vi "PSFormula_Formula Node Generation.vi"(6 "Complex Variable(T)":bool=TRUE, 10 "Var List":T1={"Names"=["d", "r"], "Types"=["Array Of Dbl", "Dbl"], "Values"=[variant(dbl[] [0.0, 1.0]), variant(dbl 5.0)]}, 11 "Fomula":string="d+((d+r)*(4+5)+7)*8") -> (0 "Error Code":i32, 3 "Formula Node":T2)   [LabVIEW 2016]
uses:
  Ctrls/PSFormula_FOR_Formula Node.ctl
  Ctrls/PSFormula_FOR_Formula Step.ctl
  Ctrls/PSFormula_FOR_Formula Para.ctl
  Ctrls/PSFormula_FOR_Formula MidVar Data.ctl
panel:
  out "Numeric":i32
  out "Fomulas In Bracket":string[](array[string])
  # "d+((d+r)*(4+5)+7)*8"
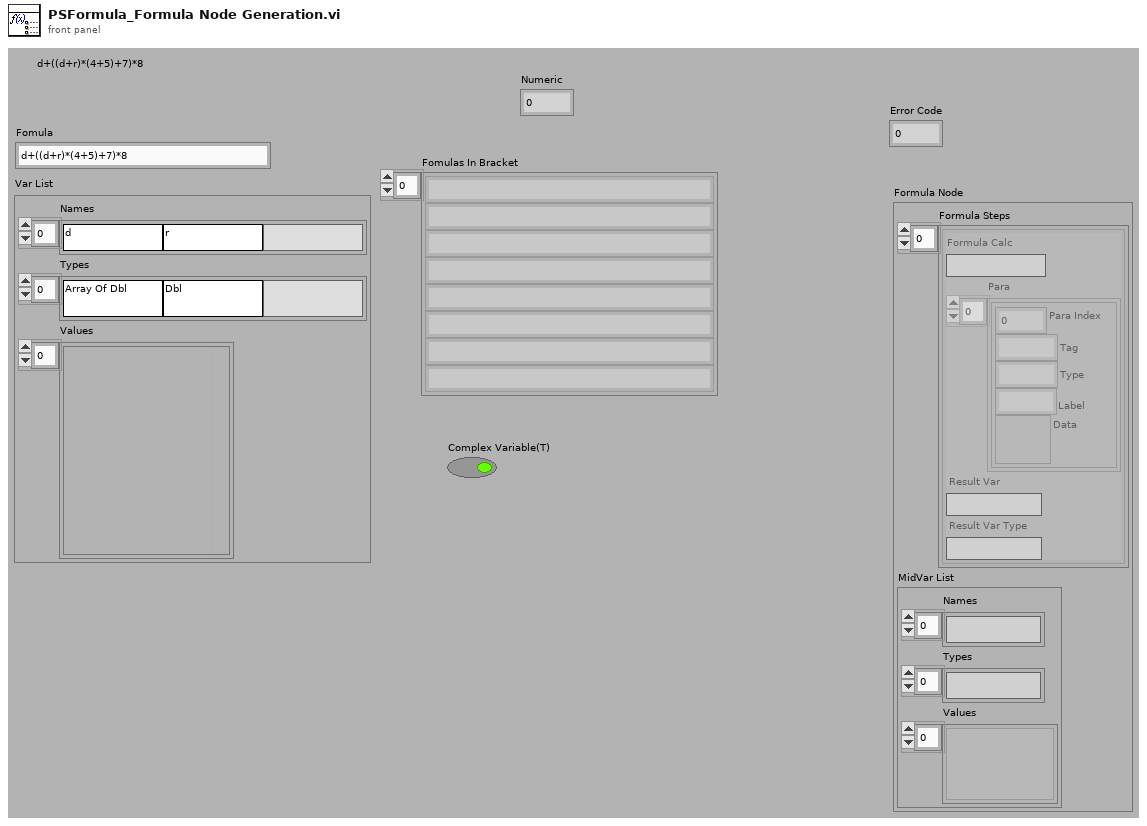
[diagram p1: front panel]
types:
  T1 = typedef "PSFormula_FOR_Formula MidVar Data.ctl" = cluster{"Names":string[], "Types":string[], "Values":variant[]}
  T2 = typedef "PSFormula_FOR_Formula Node.ctl" = cluster{"Formula Steps":T3[], "MidVar List":T1}
  T3 = typedef "PSFormula_FOR_Formula Step.ctl" = cluster{"Formula Calc":string, "Para":T4[], "Result Var":string, "Result Var Type":string}
  T4 = typedef "PSFormula_FOR_Formula Para.ctl" = cluster{"Para Index":i32, "Tag":string, "Type":string, "Label":string, "Data":variant}
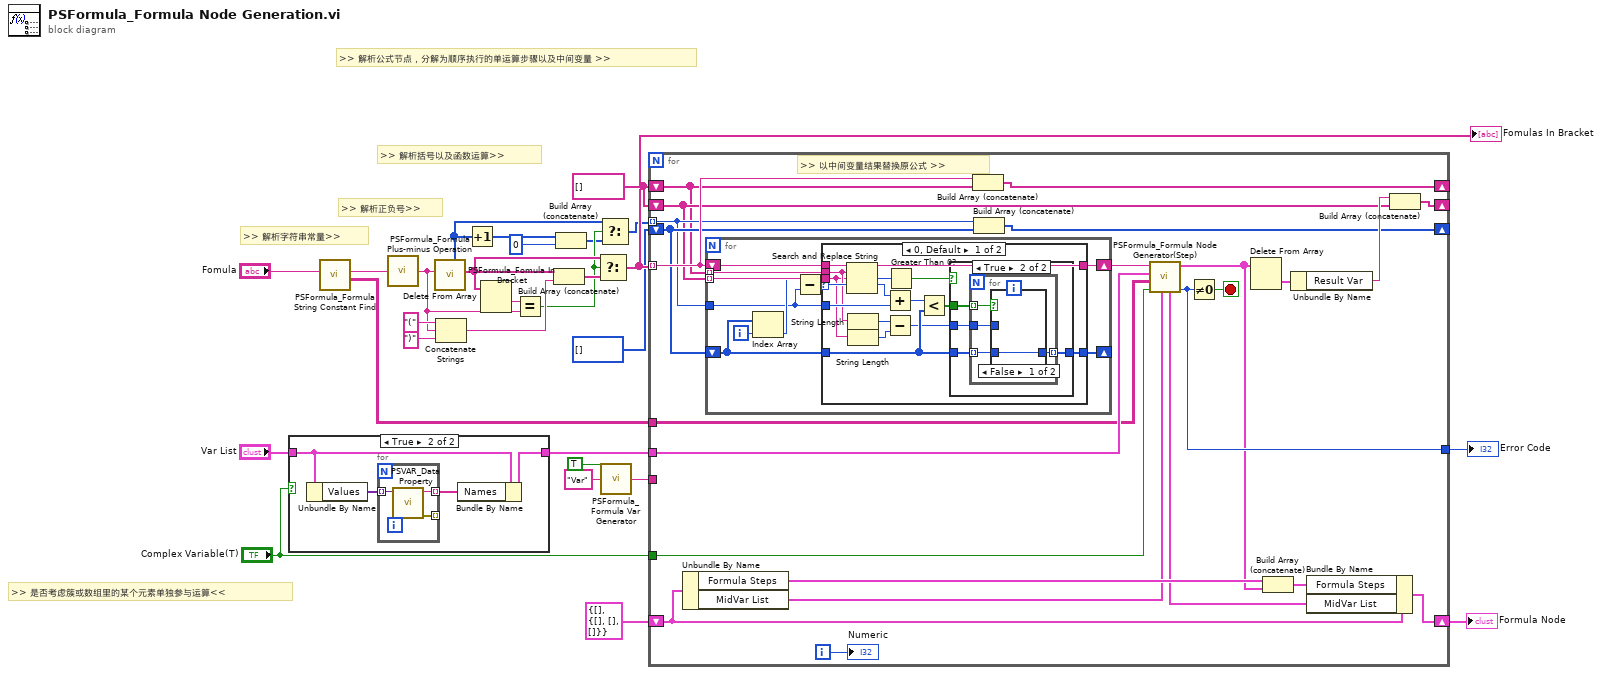
[diagram p0: block diagram]
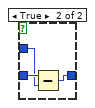
[diagram p4: hidden frame]
diagram:
  w22 = string[] []
  # ">> 是否考虑簇或数组里的某个元素单独参与运算<<"
  # ">> 解析正负号>>"
  # ">> 解析括号以及函数运算>>"
  # ">> 解析字符串常量>>"
  # ">> 解析公式节点，分解为顺序执行的单运算步骤以及中间变量 >>"
  n1 = case shown="True" "Complex Variable(T)" {
    tunnel: "Var List" -> [w29 w33]
    tunnel: [w29 w31] -> w2
    frame False {
    }
    frame True {
      n2 = Unbundle By Name(w33) -> ("Values"=w32:variant[])
      n3 = for {
        tunnel: w32 -> [w36] mode=indexing
        tunnel: [w35] -> _ mode=indexing
        tunnel: [w34] -> w30 mode=indexing
        n4 = call "PSVAR_Data Property.vi"("Data"=w36) -> ("error out"=w35:errorcluster, "Label"=w34:string)  [unwired: 6 in, 3 out]
      }
      n5 = Bundle By Name(cluster=w33, "Names"=w30) -> (w31:T1)
    }
  }
  n6 = call "PSFormula_Formula String Constant Find.vi"("Fomula"="Fomula") -> ("String Constant"=w4:string[][], "Formula"=w5:string)  [unwired: 9 in]
  n7 = call "PSFormula_Formula Plus-minus Operation.vi"("Formula"=w5) -> ("result string"=w13:string)  [unwired: 4 in]
  n8 = call "PSFormula_Fomula In Bracket.vi"("Fomula"=w13) -> ("Formulas"=w16:string[], "Position"=w10:i32[])  [unwired: 8 in, 1 out]
  n9 = Concatenate Strings("(" ("string"), w13, ")" ("string")) -> (w19:string)
  n10 = Increment(x=w10) -> (x+1=w9:i32[])
  n11 = Delete From Array(array=w16) -> (deleted portion=w18:string)  [unwired: 2 in, 1 out]
  n12 = Equal?(x=w18, y=w13) -> (x = y?=w12:bool)
  n13 = Build Array (concatenate)(w16, w19) -> (w17:string[])
  n14 = Build Array (concatenate)(w9, 0) -> (w8:i32[])
  n15 = Select(t=w16, s=w12, f=w17) -> (s? t:f=w15:string[])
  "Fomulas In Bracket" <- w15
  n16 = Select(t=w10, s=w12, f=w8) -> (s? t:f=w11:i32[])
  n17 = call "PSFormula_Formula Var Generator.vi"("Reset"=TRUE, "Formula Str"="Var") -> ("Var Next"=w23:string)  [unwired: 13 in]
  n18 = for {
    tunnel: w15 -> [w45] mode=indexing
    tunnel: w2 -> [w59]
    shift-right: [w49] -> _
    shift-left: w22 -> [w39]
    shift-right: [w54] -> w21
    shift-left: T2 {"Formula Steps"=[], "MidVar List"={"Names"=[], "Types"=[], "Values"=[]}} ("Formula Node") -> [w56]
    tunnel: w23 -> [_]
    shift-right: [w53] -> _
    shift-left: w22 -> [w40]
    tunnel: [w48] -> w20
    tunnel: w11 -> [w41] mode=indexing
    shift-right: [w43] -> _
    shift-left: i32[] [] ("Position") -> [w42]
    tunnel: w4 -> [w38]
    tunnel: "Complex Variable(T)" -> [w37]
    i -> [w44]
    stop <- w58 stop-if-true
    # ">> 以中间变量结果替换原公式 >>"
    n19 = Unbundle By Name(w56) -> ("Formula Steps"=w57:T3[], "MidVar List"=w52:T1)
    n20 = for {
      tunnel: w39 -> [w69] mode=indexing
      shift-right: [w68] -> w60
      shift-left: w45 -> [w70]
      tunnel: w40 -> [w67] mode=indexing
      shift-right: [w61] -> _
      shift-left: w42 -> [w63]
      tunnel: w41 -> [w62]
      i -> [w66]
      n21 = Index Array(array=w63, index=w66) -> (element=w65:i32)
      n22 = Subtract(x=w65, y=w62) -> (x-y=w64:i32)
      n23 = case shown="0, Default" w64 {
        selector: w64 -> [w84 _]
        tunnel: w70 -> [w86 w100]
        tunnel: w69 -> [w78 _]
        tunnel: [w85 w100] -> w68
        tunnel: w67 -> [w77 _]
        tunnel: w63 -> [w74 w101]
        tunnel: w62 -> [w81 _]
        tunnel: [w72 w101] -> w61
        frame 0, Default {
          n24 = Search and Replace String(input string=w86, search string=w78, replace string=w77, offset=w84) -> (result string=w85:string, number of replacements=w83:i32, offset past replacement=w82:i32)  [unwired: 4 in, 1 out]
          n25 = String Length(string=w78) -> (length=w76:i32)
          n26 = String Length(string=w77) -> (length=w75:i32)
          n27 = Add(x=w82, y=w81) -> (x+y=w80:i32)
          n28 = Subtract(x=w76, y=w75) -> (x-y=w73:i32)
          n29 = Greater Than 0?(x=w83) -> (x > 0?=w71:bool)
          n30 = Less?(x=w80, y=w74) -> (x < y?=w79:bool[])
          n31 = case shown="True" w71 {
            tunnel: w79 -> [_ w91]
            tunnel: w74 -> [w87 w90]
            tunnel: w73 -> [_ w89]
            tunnel: [w87 w88] -> w72
            frame False {
            }
            frame True {
              n32 = for {
                tunnel: w91 -> [w95] mode=indexing
                tunnel: w90 -> [w94] mode=indexing
                tunnel: w89 -> [w93]
                tunnel: [w92] -> w88 mode=indexing
                n33 = case shown="False" w95 {
                  tunnel: w94 -> [w96 w99]
                  tunnel: w93 -> [_ w98]
                  tunnel: [w96 w97] -> w92
                  frame False {
                  }
                  frame True {
                    n34 = Subtract(x=w99, y=w98) -> (x-y=w97:i32)
                  }
                }
              }
            }
          }
        }
        frame ..-1 {
        }
      }
    }
    n35 = Build Array (concatenate)(w45, w39) -> (w49:string[])
    n36 = Build Array (concatenate)(w41, w42) -> (w43:i32[])
    n37 = call "PSFormula_Formula Node Generator(Step).vi"("MidVar List"=w52, "Complex Variable(T)"=w37, "String Constant"=w38, "Var List"=w59, "Formula"=w60) -> ("Error Code"=w48:i32, "Formula Steps"=w47:T3[], "MidVar List"=w51:T1)  [unwired: 4 in]
    n38 = Not Equal To 0?(x=w48) -> (x != 0?=w58:bool)
    n39 = Delete From Array(array=w47) -> (deleted portion=w50:T3)  [unwired: 2 in, 1 out]
    n40 = Build Array (concatenate)(w57, w47) -> (w55:T3[])
    n41 = Unbundle By Name(w50) -> ("Result Var"=w46:string)
    n42 = Bundle By Name(cluster=w56, "Formula Steps"=w55, "MidVar List"=w51) -> (w54:T2)
    n43 = Build Array (concatenate)(w46, w40) -> (w53:string[])
    "Numeric" <- w44
  }
  "Formula Node" <- w21
  "Error Code" <- w20
